vi "Regression Metrics.vi"   [LabVIEW 2020]
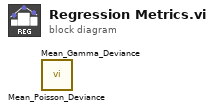
[diagram p0: block diagram]
diagram:
  n1 = call "Mean_Poisson_Deviance.vi"() -> ()  [unwired: 9 in, 3 out]
  n2 = call "Mean_Gamma_Deviance.vi"() -> ()  [unwired: 9 in, 3 out]
